vi "testcase - Convert API String to Cluster.vi"() -> ()   [LabVIEW 2017]
uses:
  df651521-38ed-47ee-a793-15e251df3308.vi
  002628dc-ed68-4010-a1bf-b76f7e223dbf.vi
  221b1020-3046-4682-8f51-ef30bd93ab5e.vi
  594a2204-1839-4150-aa7c-2fa10e07e93b.vi
  <userlib>/_NEVSTOP/Communicable State Machine(CSM)/addons/API-String-Arugments-Support/_Support/Concatenate Strings If not Empty_csm.vi
  INI-Static-Variable-Support/_Support/FlagInstance-CSMINIVariable.vi
  002628dc-ed68-4010-a1bf-b76f7e223dbf.vi/99de0c97-112a-4c86-9094-c187659127e1.vi
  <userlib>/_NEVSTOP/Communicable State Machine(CSM)/Utility/Build Error Cluster.vi
  221b1020-3046-4682-8f51-ef30bd93ab5e.vi/70cf541c-689a-4909-ae73-497058dc5e15.vi
  221b1020-3046-4682-8f51-ef30bd93ab5e.vi/9171d6c3-d5ea-4572-92dd-59f7e0660fdf.vi
  594a2204-1839-4150-aa7c-2fa10e07e93b.vi/70cf541c-689a-4909-ae73-497058dc5e15.vi
  594a2204-1839-4150-aa7c-2fa10e07e93b.vi/8441470c-f7c2-4ba6-a00e-bb382131ed64.vi
  <userlib>/_NEVSTOP/Communicable State Machine(CSM)/_Support/ChangeFlag/ChangeFlag-Read.vi
  594a2204-1839-4150-aa7c-2fa10e07e93b.vi/8441470c-f7c2-4ba6-a00e-bb382131ed64.vi/99de0c97-112a-4c86-9094-c187659127e1.vi
  <userlib>/_NEVSTOP/Communicable State Machine(CSM)/_Support/ChangeFlag/ChangeFlagDB.vi
  INI-Static-Variable-Support/_Support/CSM - Read INI String.vi
  INI-Static-Variable-Support/_Support/Populate String with INI Variable.vi
  <userlib>/_NEVSTOP/Communicable State Machine(CSM)/addons/API-String-Arugments-Support/_Support/Convert API String Arguments to Data(variant).vi
  <vilib>/Utility/Data Type/Get Type Information.vi
  <userlib>/_NEVSTOP/Communicable State Machine(CSM)/addons/API-String-Arugments-Support/_Support/Data To SingleElementsArray_csm.vi
  <userlib>/_NEVSTOP/Communicable State Machine(CSM)/addons/API-String-Arugments-Support/_Support/Data To API String Arguments.vi
  INI-Static-Variable-Support/_Support/Parse Used Session and Name.vi
  INI-Static-Variable-Support/_Support/INI-FGV(lvlibp).vi
  <userlib>/_NEVSTOP/Communicable State Machine(CSM)/addons/API-String-Arugments-Support/_Support/SingleElementsArray To Data_csm.vi
  INI-Static-Variable-Support/INI-Static-Variable-Support.lvlib
panel:
  out "cluster2":variant
  out "cluster1":variant
  out "Array":cluster{"Value":string, "Array":string[]}[](array[cluster])
  out "csm2":variant
  out "csm1":variant
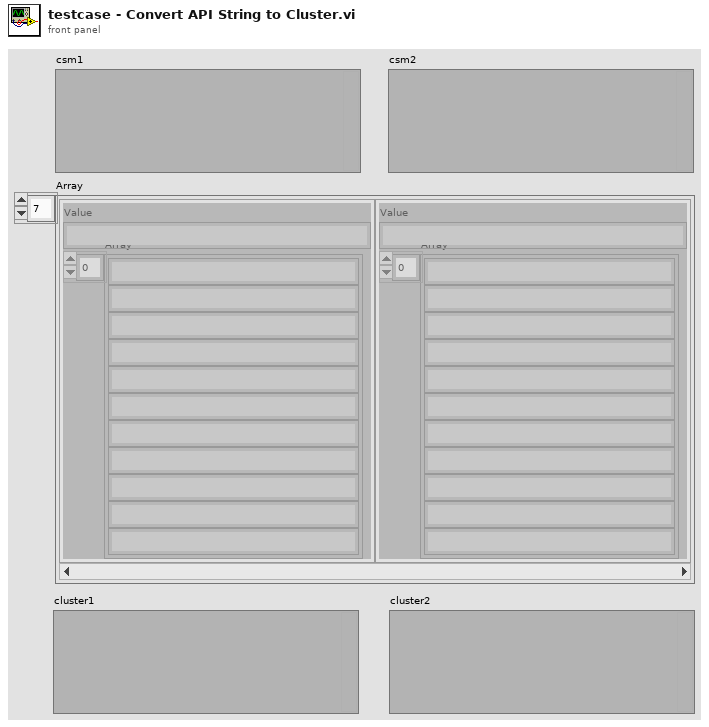
[diagram p1: front panel]
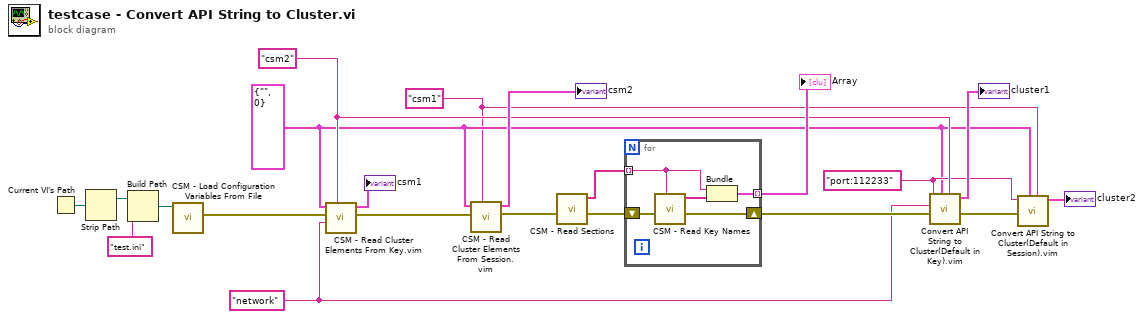
[diagram p0: block diagram]
diagram:
  w1 = "network" ("Section Name(\"\" as Default)")
  w5 = "port:112233" ("API String")
  w8 = "csm2" ("Section Name(\"\" as Default)")
  w3 = "csm1" ("Section Name(\"\" as Default)")
  w4 = cluster{"ip":string, "port":u32} {"ip"="", "port"=0}
  n1 = Current VI's Path() -> (path=w21:path)
  n2 = Strip Path(path=w21) -> (stripped path=w20:path)  [unwired: 1 out]
  n3 = Build Path(base path=w20, name or relative path="test.ini") -> (appended path=w18:path)
  n4 = call "CSM - Load Configuration Variables From File.vi"("Configuration Path"=w18) -> ("error out"=w17:errorcluster)  [unwired: 8 in]
  n5 = call "CSM - Read Cluster Elements From Key.vim"("Section Name (\"\" as Default)"=w8, "Key"=w1, "error in (no error)"=w17, "Cluster"=w4) -> ("error out"=w16:errorcluster, "Cluster out"=→"csm1":cluster{"ip":string, "port":u32})  [unwired: 3 in, 1 out]
  n6 = call "CSM - Read Cluster Elements From Session.vim"("Section Name (\"\" as Default)"=w3, "error in (no error)"=w16, "Cluster"=w4) -> ("error out"=w10:errorcluster, "Cluster out"=→"csm2":cluster{"ip":string, "port":u32})  [unwired: 5 in]
  n7 = call "CSM - Read Sections.vi"("error in (no error)"=w10) -> ("error out"=w13:errorcluster, "Sections"=w12:string[])  [unwired: 7 in]
  n8 = for {
    tunnel: w12 -> [w23] mode=indexing
    tunnel: [w24] -> w11 mode=indexing
    shift-right: [w22] -> w9
    shift-left: w13 -> [w26]
    n9 = call "CSM - Read Key Names.vi"("Section Name (\"\" as Default)"=w23, "error in (no error)"=w26) -> ("error out"=w22:errorcluster, "Keys"=w25:string[])  [unwired: 6 in]
    n10 = Bundle("Value"=w23, "Keys"=w25) -> (w24:cluster{"Value":string, "Keys":string[]})  [unwired: 1 in]
  }
  "Array" <- w11
  n11 = call "Convert API String to Cluster(Default in Key).vim"("Section Name(\"\" as Default)"=w8, "Type"=w4, "error in (no error)"=w9, "Variable Name"=w1, "API String"=w5) -> ("error"=w6:errorcluster, "Data"=→"cluster1":cluster{"ip":string, "port":u32})  [unwired: 5 in]
  n12 = call "Convert API String to Cluster(Default in Session).vim"("Section Name(\"\" as Default)"=w3, "Type"=w4, "error in (no error)"=w6, "API String"=w5) -> ("Data"=→"cluster2":cluster{"ip":string, "port":u32})  [unwired: 6 in, 1 out]
